vi "Build Measurement Array.vi"() -> ()   [LabVIEW 2018]
panel:
  in  "Reset":bool
  out "Counter":u16
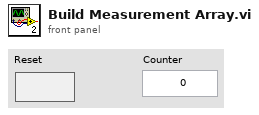
[diagram p1: front panel]
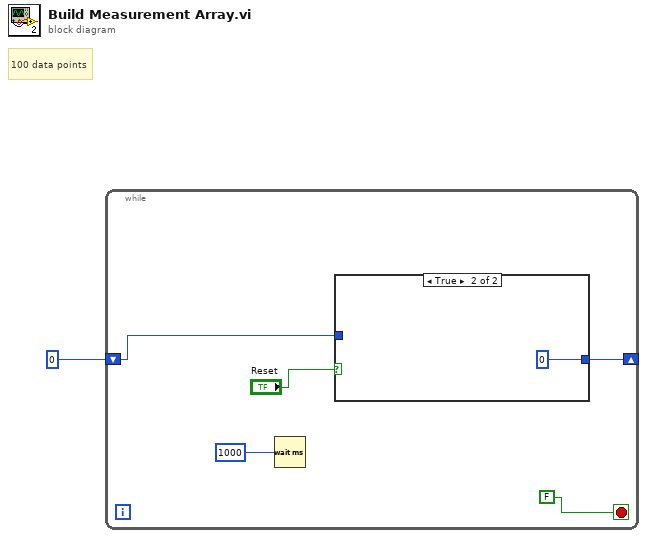
[diagram p0: block diagram]
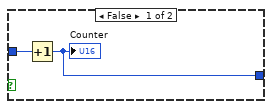
[diagram p2: hidden frame]
diagram:
  # "100 data points"
  n1 = while {
    shift-right: [w5] -> _
    shift-left: 0 -> [w4]
    stop <- FALSE stop-if-true
    n2 = Wait (ms)(milliseconds to wait=1000) -> ()  [unwired: 1 out]
    n3 = case shown="True" "Reset" {
      tunnel: [w8 0] -> w5
      tunnel: w4 -> [w7 _]
      frame False {
        n4 = Increment(x=w7) -> (x+1=w8:i32)
        "Counter" <- w8
      }
      frame True {
      }
    }
  }
